vi "update.vi"(7 "Pressure":dbl, 8 "error in (no error)":errorcluster, 9 "Humidity":dbl, 10 "Temperature":dbl, 11 "StatisticsDisplay.lvclass":refnum<class "StatisticsDisplay.lvclass">) -> (0 "error out":errorcluster, 3 "StatisticsDisplay.lvclass 2":refnum<class "StatisticsDisplay.lvclass">)   [LabVIEW 2020, in "StatisticsDisplay.lvclass"]
uses:
  StatisticsDisplay.lvclass
  StatisticsDisplay.lvclass/StatisticsDisplay.ctl
panel:
  # "Connector Pane"
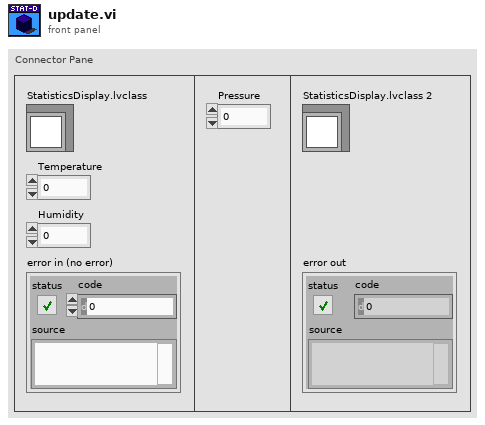
[diagram p1: front panel]
types:
  T1 = typedef "StatisticsDisplay.lvclass/StatisticsData.ctl" = cluster{"maxTemp":dbl, "minTemp":dbl, "TempSum":dbl, "nReadings":i32}
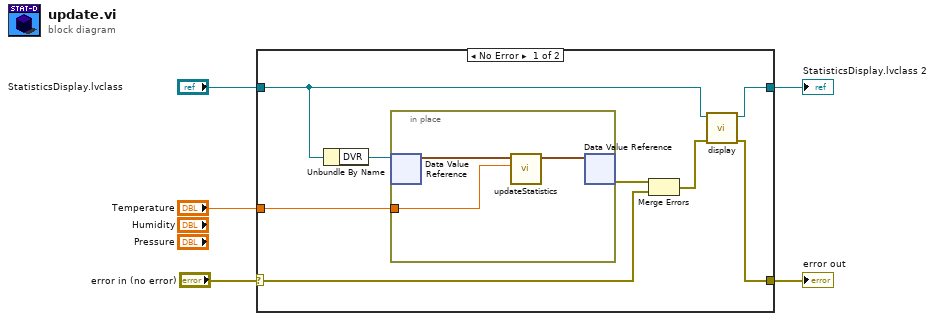
[diagram p0: block diagram]
diagram:
  n1 = case shown="No Error" "error in (no error)" {
    selector: "error in (no error)" -> [w13 w17]
    tunnel: [w12 w17] -> w4
    tunnel: [w11 w18] -> w3
    tunnel: "Temperature" -> [w9 _]
    tunnel: "StatisticsDisplay.lvclass" -> [w8 w18]
    frame No Error {
      n2 = Unbundle By Name(w8) -> ("DVR"=w10:refnum<data-value>)
      n3 = in-place {
        in-place-border: w9 -> [w14]
        n4 = in-place-dvr #1(w10) -> (w16:T1)  [unwired: 1 out]
        n5 = call "updateStatistics.vi"("Temperature"=w14, "StatisticsData in"=w16) -> ("StatisticsData out"=w15:T1)  [unwired: 9 in]
        n6 = in-place-dvr #1(w15) -> (w6:errorcluster)  [unwired: 1 out]
      }
      n7 = Merge Errors(w6, w13) -> (w7:errorcluster)
      n8 = call-dynamic "display.vi"("error in (no error)"=w7, "Display"=w8) -> ("error out"=w12:errorcluster, "CurrentConditionsDisplay.lvclass 2"=w11:refnum<class "StatisticsDisplay.lvclass">)  [unwired: 8 in]
    }
    frame Error {
    }
  }
  "StatisticsDisplay.lvclass 2" <- w3
  "error out" <- w4
